vi "initialise the FTR Selection.vi"(6 "Local Data in":T2, 7 "UI Refs":T1, 8 "error in (no error)":errorcluster) -> (0 "error out":errorcluster)   [LabVIEW 2024]
uses:
  Controls/RVHR - Local Data.ctl
  Controls/Test Cluster.ctl
  Controls/Excluded Information.ctl
  Controls/Language.ctl
  Controls/Device_Type.ctl
  <vilib>/Utility/miscctls.llb/LVRectTypeDef.ctl
  <vilib>/Utility/miscctls.llb/LVBoundsTypeDef.ctl
  Controls/RVHR - UI Refs.ctl
  Controls/Run Listbox Command.ctl
  Controls/DB Manager Commands.ctl
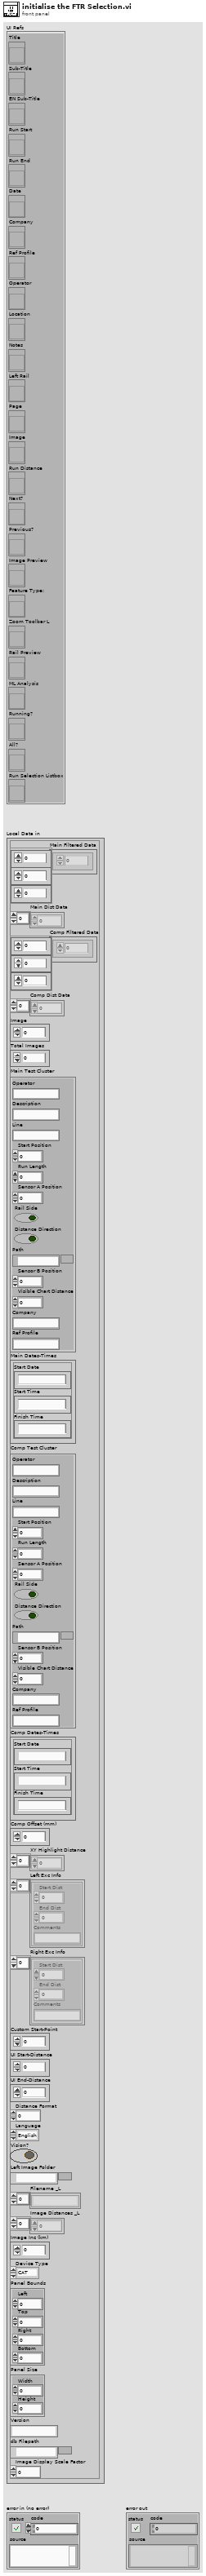
[diagram p1: front panel]
types:
  T1 = typedef "RVHR - UI Refs.ctl" = cluster{"Title":refnum<vi>, "Sub-Title":refnum<vi>, "EN Sub-Title":refnum<vi>, "Run Start":refnum<vi>, "Run End":refnum<vi>, "Date":refnum<vi>, "Company":refnum<vi>, "Ref Profile":refnum<vi>, "Operator":refnum<vi>, "Location":refnum<vi>, "Notes":refnum<vi>, "Left Rail":refnum<vi>, "Page":refnum<vi>, "Image":refnum<vi>, "Run Distance":refnum<vi>, "Next?":refnum<vi>, "Previous?":refnum<vi>, "Image Preview":refnum<vi>, "Feature Type:":refnum<vi>, "Zoom Toolbar L":refnum<vi>, "Rail Preview":refnum<vi>, "ML Analysis":refnum<vi>, "Running?":refnum<vi>, "All?":refnum<vi>, "Run Selection Listbox":refnum<vi>}
  T2 = typedef "RVHR - Local Data.ctl" = cluster{"Main Filtered Data":dbl[][][], "Main Dist Data":dbl[], "Comp Filtered Data":dbl[][][], "Comp Dist Data":dbl[], "Image":u16, "Total Images":u16, "Main Test Cluster":T3, "Main Dates-Times":cluster{"Start Date":string, "Start Time":string, "Finish Time":string}, "Comp Test Cluster":T3, "Comp Dates-Times":cluster{"Start Date":string, "Start Time":string, "Finish Time":string}, "Comp Offset (mm)":i64, "XY Highlight Distance":dbl[], "Left Exc Info":T4[], "Right Exc Info":T4[], "Custom Start-Point":dbl, "UI Start-Distance":dbl, "UI End-Distance":dbl, "Distance Format":u8, "Language":T5, "Vision?":bool, "Left Image Folder":path, "Filename _L":string[], "Image Distances _L":dbl[], "Image Inc (km)":dbl, "Device Type":T6, "Panel Bounds":T7, "Panel Size":T8, "Version":string, "db Filepath":path, "Image Display Scale Factor":dbl}
  T3 = typedef "Test Cluster.ctl" = cluster{"Operator":string, "Description":string, "Line":string, "Start Position":dbl, "Run Length":dbl, "Sensor A Position":dbl, "Rail Side":bool, "Distance Direction":bool, "Path":path, "Sensor B Position":dbl, "Visible Chart Distance":dbl, "Company":string, "Ref Profile":string}
  T4 = typedef "Excluded Information.ctl" = cluster{"Start Dist":dbl, "End Dist":dbl, "Comments":string}
  T5 = typedef "Language.ctl" = enum16{"English", "Chinese", "German"}
  T6 = typedef "Device_Type.ctl" = enum16{"CAT", "Bi-CAT", "YRCA", "RCA", "RV-HR", "TV-HR"}
  T7 = typedef "LVRectTypeDef.ctl" = cluster{"Left":i16, "Top":i16, "Right":i16, "Bottom":i16}
  T8 = typedef "LVBoundsTypeDef.ctl" = cluster{"Width":u32, "Height":u32}
  T9 = typedef "DB Manager Commands.ctl" = enum16{"Get Image", "Get Preview", "Add", "Remove", "Update", "Get FTR Names"}
  T10 = typedef "Run Listbox Command.ctl" = enum16{"Init", "Item Names", "Update", "Update All", "Get Selections", "Clear"}
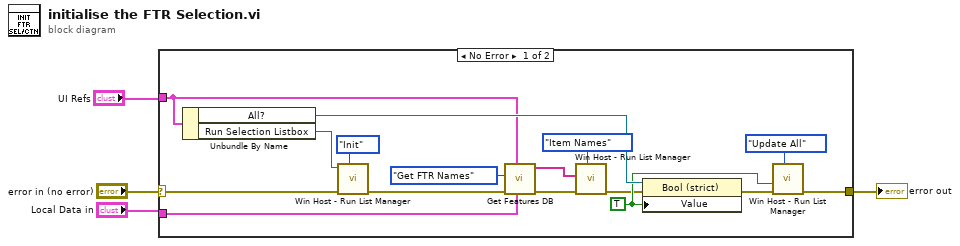
[diagram p0: block diagram]
diagram:
  n1 = case shown="No Error" "error in (no error)" {
    selector: "error in (no error)" -> [w20 w21]
    tunnel: [w14 w21] -> w2
    tunnel: "UI Refs" -> [w6 _]
    tunnel: "Local Data in" -> [w7 _]
    frame No Error {
      w13 = TRUE ("Value")
      n2 = Unbundle By Name(w6) -> ("All?"=w17:refnum<vi>, "Run Selection Listbox"=w18:refnum<vi>)
      n3 = call "Win Host - Run List Manager.vi"("Command"=Run_Listbox_Command."Init", "error in (no error)"=w20, "ListBox in"=w18) -> ("error out"=w8:errorcluster)  [unwired: 5 in, 3 out]
      n4 = call "Get Features DB.vi"("Local Data in"=w7, "UI References"=w6, "error in (no error)"=w8, "Action"=DB_Manager_Commands."Get FTR Names") -> ("error out"=w9:errorcluster, "FTR Names"=w5:string[])  [unwired: 3 in, 3 out]
      n5 = call "Win Host - Run List Manager.vi"("Command"=Run_Listbox_Command."Item Names", "error in (no error)"=w9, "Item Names"=w5) -> ("error out"=w11:errorcluster)  [unwired: 5 in, 3 out]
      n6 = property class="Bool (strict)"(reference=w17, error in=w11, "Value"=w13) -> (error out=w15:errorcluster)  [unwired: 1 out]
      n7 = call "Win Host - Run List Manager.vi"("Command"=Run_Listbox_Command."Update All", "error in (no error)"=w15, "All? IN"=w13) -> ("error out"=w14:errorcluster)  [unwired: 5 in, 3 out]
    }
    frame Error {
    }
  }
  "error out" <- w2
